vi "Auto_Routine_DepositBalance.vi"(8 "error in (no error)":errorcluster) -> (0 "error out":errorcluster)   [LabVIEW 2020]
doc: "Deposites a cone on the upper node then balances\nInputs:\n--ErrorIn--\nOutputs:\n--ErrorOut--"
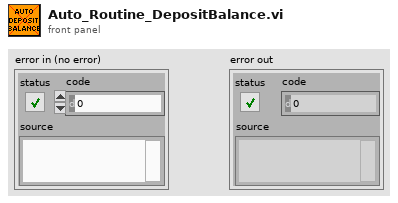
[diagram p1: front panel]
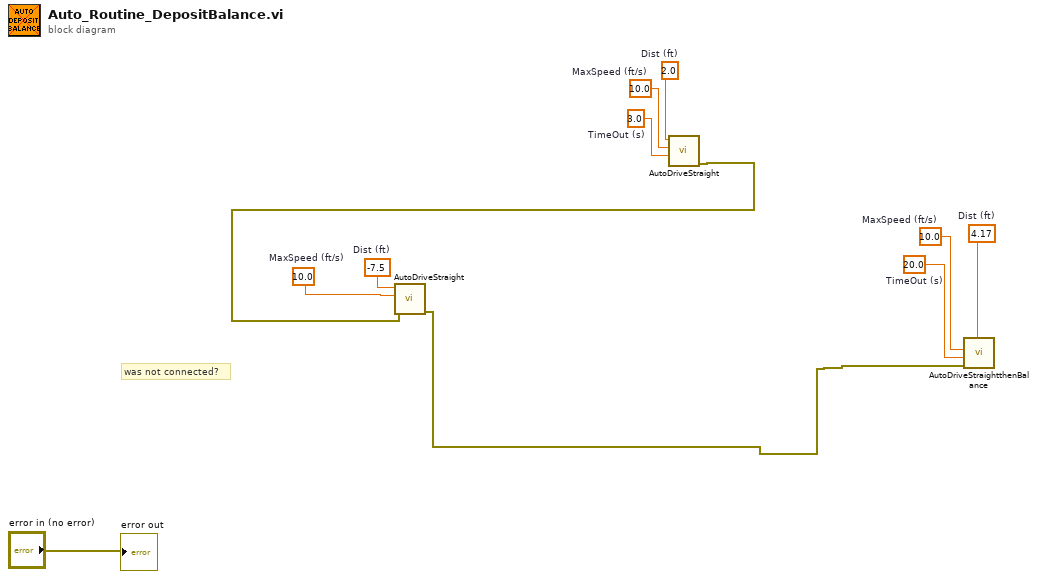
[diagram p0: block diagram]
diagram:
  w8 = 20.0  # TimeOut (s)
  w7 = 4.17  # Dist (ft)
  w6 = 10.0  # MaxSpeed (ft/s)
  w5 = 10.0  # MaxSpeed (ft/s)
  w11 = 3.0  # TimeOut (s)
  w10 = 10.0  # MaxSpeed (ft/s)
  w9 = 2.0  # Dist (ft)
  w4 = -7.5  # Dist (ft)
  # "was not connected?"
  n1 = call "AutoDriveStraight.vi"("TimeOut (s)"=w11, "MaxSpeed (ft/s)"=w10, "Dist (ft)"=w9) -> ("error out"=w2:errorcluster)  [unwired: 8 in]
  n2 = call "AutoDriveStraight.vi"("error in (no error)"=w2, "MaxSpeed (ft/s)"=w5, "Dist (ft)"=w4) -> ("error out"=w1:errorcluster)  [unwired: 8 in]
  n3 = call "AutoDriveStraightthenBalance.vi"("error in (no error)"=w1, "TimeOut (s)"=w8, "MaxSpeed (ft/s)"=w6, "Dist (ft)"=w7) -> ()  [unwired: 7 in, 1 out]
  "error out" <- "error in (no error)"
